vi "Variable list Stroker digital.vi"() -> (6 "Variant":variant, 10 "Array":T1[](array[typedef]))   [LabVIEW 2011]
uses:
  Measurments Handling/Fixed Digital Channel Definition.ctl
  Measurments Handling/Update frequensies.ctl
  Measurments Handling/Channel catagory Enum.ctl
  Variable List Stroker Digital.ctl
  <vilib>/Utility/VariantDataType/GetNumericInfo.vi
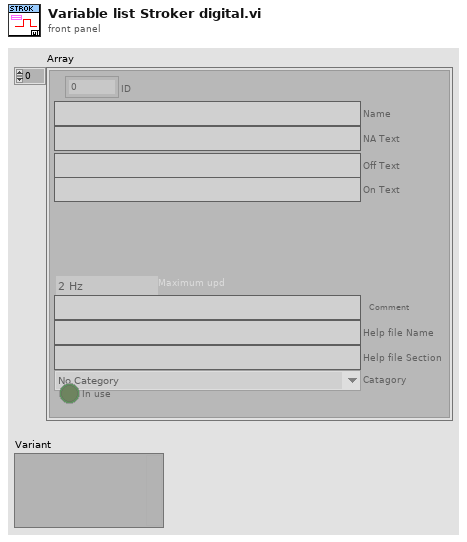
[diagram p1: front panel]
types:
  T1 = typedef "Fixed Digital Channel Definition.ctl" = cluster{"ID":u16, "Name":string, "NA Text":string, "Off Text":string, "On Text":string, "Maximum upd":T2, "Comment":string, "Help file Name":string, "Help file Section ":string, "Catagory":T3, "In use":bool}
  T2 = typedef "Update frequensies.ctl" = enum16{"2 Hz", "1 Hz", "0.1 Hz"}
  T3 = typedef "Channel catagory Enum.ctl" = enum16{"No Category", "Power", "Temperature", "Pressure"}
  T4 = typedef "Variable List Stroker Digital.ctl" = enum16{"Tool Stroke enable Valve", "Tool Stroke direction Valve", "Tool Anchor Valve", "Tool Relay 1", "Tool Relay 2", "Tool node pressure 1", "Tool node pressure 2", "Tool node solenoid", "Tool High G Monitoring", "Tool High G Recording", "Tool High G Data ready", "Tool Anchor(Not Available)", "Tool error Controller", "Tool error Pressure 1", "Tool error Pressure 2", "Tool error Solenoid", "Tool error Upper Tension Sub", "Tool error Lower Tension Sub", "Tool stopped Controller", "Tool stopped Pressure 1", "Tool stopped Pressure 2", "Tool stopped Solenoid", "Stroke Target seeking", "Stroke Moving Out", "Stroke Moving Inn", "Stroke valves set for Out", "Stroke valves set for In", "Stroke In (force)", "Stroke Out (force)", "Stroke Force decreasing(in)", "Stroke Force decreasing(out)", "Stroke Force change not correct", "Stroke SLIPS established P1", "Stroke SLIPS established P2", "Stroke SLIPS established", "Stroke Pressure Monitor Ongoing", "Stroke Pressure Monitor Ending", "Stroke Upper Tension Sub", "Stroke Lower Tension Sub"}
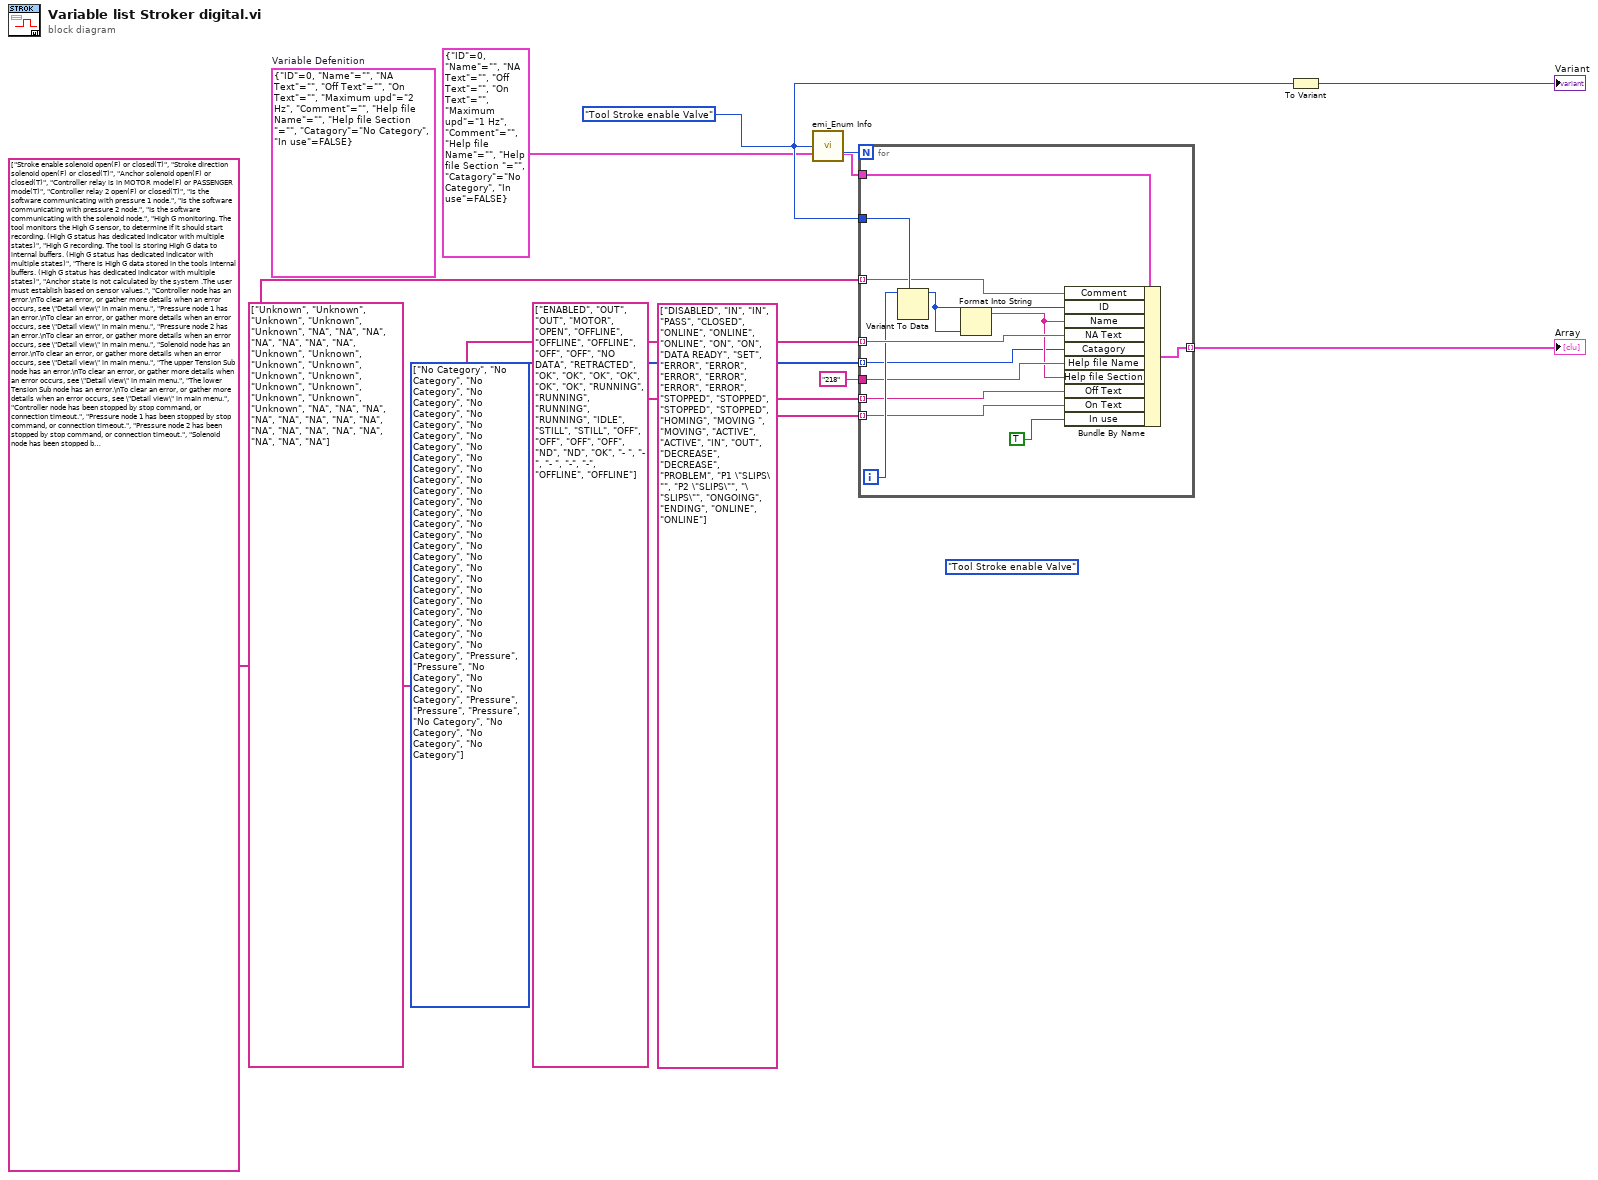
[diagram p0: block diagram]
diagram:
  (unwired) Variable_List_Stroker_Digital."Tool Stroke enable Valve" ("Action")
  (unwired) T1 {"ID"=0, "Name"="", "NA Text"="", "Off Text"="", "On Text"="", "Maximum upd"=enum."2 Hz", "Comment"="", "Help file Name"="", "Help file Section "="", "Catagory"=enum."No Category", "In use"=FALSE}  # Variable Defenition
  w5 = T3[] [enum."No Category", enum."No Category", enum."No Category", enum."No Category", enum."No Category", enum."No Category", enum."No Category", enum."No Category", enum."No Category", enum."No Category", enum."No Category", enum."No Category", enum."No Category", enum."No Category", enum."No Category", enum."No Category", enum."No Category", enum."No Category", enum."No Category", enum."No Category", enum."No Category", enum."No Category", enum."No Category", enum."No Category", enum."No Category", enum."No Category", enum."No Category", enum."Pressure", enum."Pressure", enum."No Category", enum."No Category", enum."No Category", enum."Pressure", enum."Pressure", enum."Pressure", enum."No Category", enum."No Category", enum."No Category", enum."No Category"] items=["No Category", "Power", "Temperature", "Pressure"]
  w9 = Variable_List_Stroker_Digital."Tool Stroke enable Valve" ("Action")
  n1 = call "emi_Enum Info.vi"("Enum"=w9) -> ("Numb Elements"=w2:i32)  [unwired: 11 in, 3 out]
  n2 = for {
    N: w2 -> [_]
    tunnel: w9 -> [w24]
    tunnel: T1 {"ID"=0, "Name"="", "NA Text"="", "Off Text"="", "On Text"="", "Maximum upd"=enum."1 Hz", "Comment"="", "Help file Name"="", "Help file Section "="", "Catagory"=enum."No Category", "In use"=FALSE} ("Variable Defenition") -> [w21]
    tunnel: [w22] -> w10 mode=indexing
    tunnel: string[] ["Unknown", "Unknown", "Unknown", "Unknown", "Unknown", "NA", "NA", "NA", "NA", "NA", "NA", "NA", "Unknown", "Unknown", "Unknown", "Unknown", "Unknown", "Unknown", "Unknown", "Unknown", "Unknown", "Unknown", "Unknown", "NA", "NA", "NA", "NA", "NA", "NA", "NA", "NA", "NA", "NA", "NA", "NA", "NA", "NA", "NA", "NA"] -> [w20] mode=indexing
    tunnel: w5 -> [w16] mode=indexing
    tunnel: "218" -> [w18]
    tunnel: string[] ["ENABLED", "OUT", "OUT", "MOTOR", "OPEN", "OFFLINE", "OFFLINE", "OFFLINE", "OFF", "OFF", "NO DATA", "RETRACTED", "OK", "OK", "OK", "OK", "OK", "OK", "RUNNING", "RUNNING", "RUNNING", "RUNNING", "IDLE", "STILL", "STILL", "OFF", "OFF", "OFF", "OFF", "ND", "ND", "OK", "- ", "- ", "- ", "-", "-", "OFFLINE", "OFFLINE"] -> [w15] mode=indexing
    tunnel: string[] ["DISABLED", "IN", "IN", "PASS", "CLOSED", "ONLINE", "ONLINE", "ONLINE", "ON", "ON", "DATA READY", "SET", "ERROR", "ERROR", "ERROR", "ERROR", "ERROR", "ERROR", "STOPPED", "STOPPED", "STOPPED", "STOPPED", "HOMING", "MOVING ", "MOVING", "ACTIVE", "ACTIVE", "IN", "OUT", "DECREASE", "DECREASE", "PROBLEM", "P1 \"SLIPS\"", "P2 \"SLIPS\"", "\"SLIPS\"", "ONGOING", "ENDING", "ONLINE", "ONLINE"] -> [w14] mode=indexing
    tunnel: string[] ["Stroke enable solenoid open(F) or closed(T)", "Stroke direction solenoid open(F) or closed(T)", "Anchor solenoid open(F) or closed(T)", "Controller relay is in MOTOR mode(F) or PASSENGER mode(T)", "Controller relay 2 open(F) or closed(T)", "Is the software communicating with pressure 1 node.", "Is the software communicating with pressure 2 node.", "Is the software communicating with the solenoid node.", "High G monitoring. The tool monitors the High G sensor, to determine if it should start recording. (High G status has dedicated indicator with multiple states)", "High G recording. The tool is storing High G data to internal buffers. (High G status has dedicated indicator with multiple states)", "There is High G data stored in the tools internal buffers. (High G status has dedicated indicator with multiple states)", "Anchor state is not calculated by the system .The user must establish based on sensor values.", "Controller node has an error.\nTo clear an error, or gather more details when an error occurs, see \"Detail view\" in main menu.", "Pressure node 1 has an error.\nTo clear an error, or gather more details when an error occurs, see \"Detail view\" in main menu.", "Pressure node 2 has an error.\nTo clear an error, or gather more details when an error occurs, see \"Detail view\" in main menu.", "Solenoid node has an error.\nTo clear an error, or gather more details when an error occurs, see \"Detail view\" in main menu.", "The upper Tension Sub node has an error.\nTo clear an error, or gather more details when an error occurs, see \"Detail view\" in main menu.", "The lower Tension Sub node has an error.\nTo clear an error, or gather more details when an error occurs, see \"Detail view\" in main menu.", "Controller node has been stopped by stop command, or connection timeout.", "Pressure node 1 has been stopped by stop command, or connection timeout.", "Pressure node 2 has been stopped by stop command, or connection timeout.", "Solenoid node has been stopped by stop command, or connection timeout.", "Tool stroke is moving to a preset mm target. This should be the result of a \"Go to\" command. ", "Stroke has been detected as moving out based on position data over time", "Stroke has been detected as moving in based on position data over time", "Stroke hydraulic valves are positioned to move the stroke out.", "Stroke hydraulic valves are positioned to move the stroke in.", "Pressure readings are indicating that the stroke is moving in", "Pressure readings are indicating that the stroke is moving out", "Pressure readings are indicating that the inward stroke force is decreasing. ", "Pressure readings are indicating that the outward stroke force is decreasing. ", "Stroke force is decreasing when it should be increasing. \nExpected: When pressure is over limit to indicate movement, and valves are set for movement, the pressure on the stroking side is not expected to fall.", "Pressure node 1 indicates that SLIPS has been established.", "Pressure node 2 indicates that SLIPS has been established.", "Both pressure nodes indicate that SLIPS has been established.", "Pressure monitoring state.", "Pressure monitoring shutting down. Should never be active for long periods.", "Is the software communicating with the upper tension sub node?", "Is the software communicating with the lower tension sub node."] -> [w13] mode=indexing
    i -> [w19]
    n3 = Variant To Data(type=w24, Variant=w19) -> (data=w23:T4)  [unwired: 1 in, 1 out]
    n4 = Format Into String(w23) -> (resulting string=w17:string)  [unwired: 3 in, 1 out]
    n5 = Bundle By Name(cluster=w21, "Comment"=w13, "ID"=w23, "Name"=w17, "NA Text"=w20, "Catagory"=w16, "Help file Name"=w18, "Help file Section"=w17, "Off Text"=w15, "On Text"=w14, "In use"=TRUE) -> (w22:T1)
  }
  "Array" <- w10
  n6 = To Variant(anything=w9) -> (Variant=→"Variant":variant)
